vi "system.DSP.runCalculation.vi"(8 "error in (no error)":errorcluster, 10 "DSP.runCalculation":T1 {"runCalculation"."runCalculation"."FFT config"."export mode" items=["Power Spectrum", "Power Spectral Density"]; "runCalculation"."runCalculation"."FFT config"."window" items=["Rectangle"=0, "Hanning"=1, "Hamming"=2, "Blackman-Harris"=3, "Exact Blackman"=4, "Blackman"=5, "Flat Top"=6, "4 Term B-Harris "=7, "7 Term B-Harris"=8, "Low Sidelobe"=9, "Blackman Nuttall"=11, "Triangle"=30, "Bartlett-Hanning"=31, "Bohman"=32, "Parzen"=33, "Welch"=34, "Kaiser"=60, "Dolph-Chebyshev"=61, "Gaussian"=62]; "runCalculation"."runCalculation"."FFT config"."averaging parameters"."number of averages" min=1; "runCalculation"."runCalculation"."Lockin config"."TC (s)" format="%#_13g"}, 11 "system":refnum<class "multichannel-lockin.lvclass">) -> (0 "error out":errorcluster, 3 "system out":refnum<class "multichannel-lockin.lvclass">)   [LabVIEW 2019, in "multichannel-lockin.lvclass"]
doc: "---------------------------------------------------------------\nJKI State Machine Objects™\nhttp://jki.net/state-machine-objects/\nCopyright (C) 2005-2015, JKI <info@jki.net>\nALL RIGHTS RESERVEDJKI State Machine Objects (SMO) 1.0.0.4\nJKI - JKI\nCopyright (c) 2015, JKI"
uses:
  multichannel-lockin.lvclass
  Typedefs/PrivateEvents--system.DSP.runCalculation.ctl
  DSP/Typedefs/PrivateEvents--DSP.RunCalculation.ctl
  DSP/Typedefs/LP_Config.ctl
  DSP.lockin/Typedefs/Lockin_Config.ctl
  DSP/Typedefs/FFT_Config.ctl
  <vilib>/Analysis/4window.llb/windowTd.ctl
  <vilib>/measure/maspectr.llb/Power Spectrum and PSD Export Mode.ctl
  multichannel-lockin.lvclass/multichannel-lockin.ctl
  DSP/DSP.lvclass
  DSP.lockin/DSP_lockin.lvclass
  <vilib>/Analysis/NI_AALPro.lvlib
  <vilib>/measure/NI_MAPro.lvlib
panel:
  # "For instructions on how to use the JKI State Machine Objects, examples and video tutorials, visit:\nhttp://jki.net/state-machine-objects/\n\nJKI State Machine Objects™\nhttp://jki.net/state-machine-objects/\nCopyright (C) 2005-2015, JKI <info@jki.net>\nALL RIGHTS RESERVED"
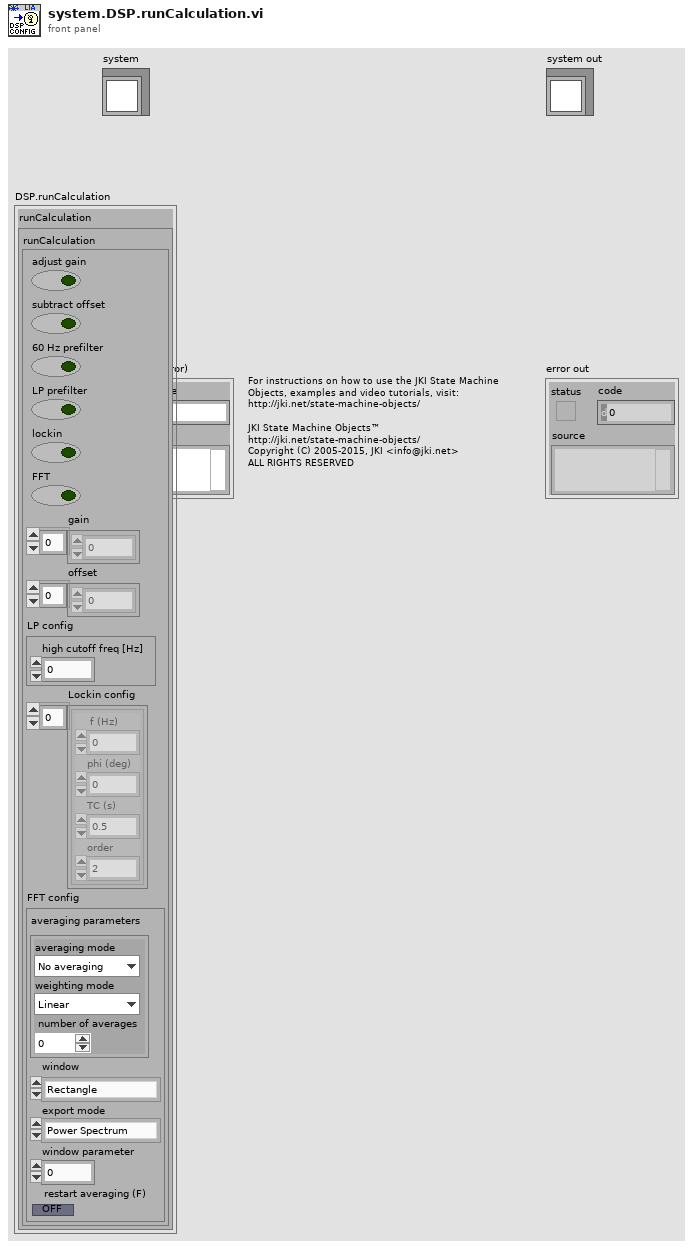
[diagram p1: front panel]
types:
  T1 = typedef "multichannel-lockin.lvclass/PrivateEvents--system.DSP.runCalculation.ctl" = cluster{"runCalculation":T2}
  T2 = typedef "DSP.lvclass/PrivateEvents--DSP.RunCalculation.ctl" = cluster{"runCalculation":cluster{"adjust gain":bool, "subtract offset":bool, "60 Hz prefilter":bool, "LP prefilter":bool, "lockin":bool, "FFT":bool, "gain":dbl[], "offset":dbl[], "LP config":T3, "Lockin config":T4, "FFT config":T5}}
  T3 = typedef "DSP.lvclass/LP_Config.ctl" = cluster{"high cutoff freq [Hz]":dbl}
  T4 = typedef "DSP_lockin.lvclass/Lockin_Config.ctl" = cluster{" f (Hz)":dbl, "phi (deg)":dbl, "TC (s)":dbl, "order":i32}[]
  T5 = typedef "DSP.lvclass/FFT_Config.ctl" = cluster{"averaging parameters":cluster{"averaging mode":enum16{"No averaging", "Vector averaging", "RMS averaging", "Peak hold"}, "weighting mode":enum16{"Linear", "Exponential"}, "number of averages":u32}, "window":T6, "export mode":T7, "window parameter":dbl, "restart averaging (F)":bool}
  T6 = typedef "NI_AALPro.lvlib/windowTd.ctl" = u32
  T7 = typedef "NI_MAPro.lvlib/Power Spectrum and PSD Export Mode.ctl" = u16
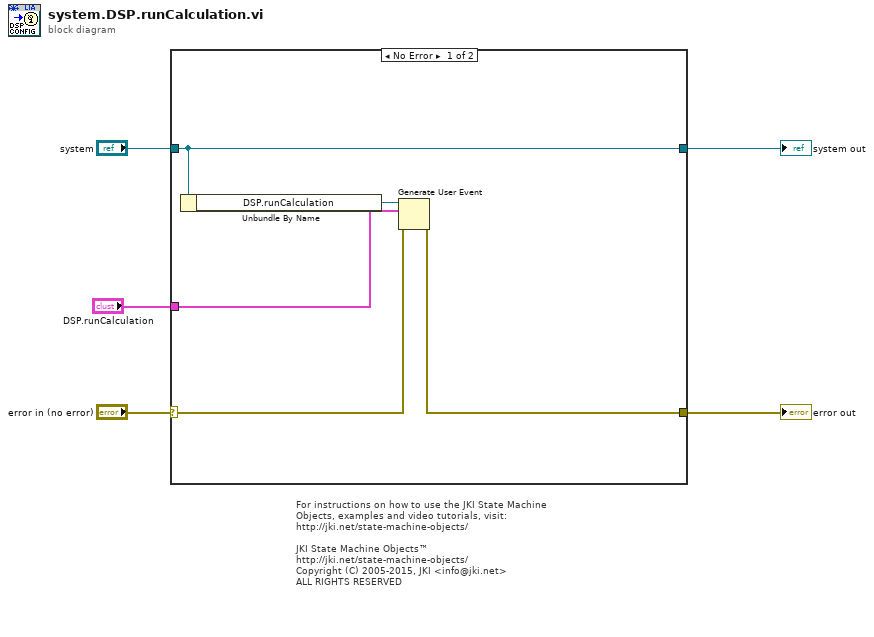
[diagram p0: block diagram]
diagram:
  # "For instructions on how to use the JKI State Machine Objects, examples and video tutorials, visit:\nhttp://jki.net/state-machine-objects/\n\nJKI State Machine Objects™\nhttp://jki.net/state-machine-objects/\nCopyright (C) 2005-2015, JKI <info@jki.net>\nALL RIGHTS RESERVED"
  n1 = case shown="No Error" "error in (no error)" {
    selector: "error in (no error)" -> [w10 w12]
    tunnel: [w7 w12] -> w4
    tunnel: [w6 w11] -> w5
    tunnel: "system" -> [w6 w11]
    tunnel: "DSP.runCalculation" -> [w9 _]
    frame No Error {
      n2 = Unbundle By Name(w6) -> ("DSP.runCalculation"=w8:refnum<user-event>)
      n3 = Generate User Event(user event=w8, event data cluster=w9, error in=w10) -> (error out=w7:errorcluster)  [unwired: 1 in, 1 out]
    }
    frame Error {
    }
  }
  "error out" <- w4
  "system out" <- w5
